vi "Poll Data.vi"(8 "error in":errorcluster, 11 "CR5 in":refnum<class "CR5.lvclass">) -> (0 "error out":errorcluster, 2 "Data Out":refnum<class "Data.lvclass">, 3 "CR5 out":refnum<class "CR5.lvclass">)   [LabVIEW 2015, in "CR5.lvclass"]
doc: "Use this VI when the hygrometer has been set to poll to poll data from the device. The hygrometer is set to poll via commands at boot time."
uses:
  CR5.lvclass
  Reusable/Data/Data.lvclass
  Reusable/Session APIs/Serial/Serial Session.lvclass
  CR5.lvclass/CR5.ctl
  Data/CR5 Data.lvclass
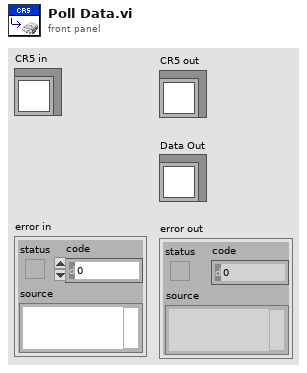
[diagram p1: front panel]
types:
  T1 = typedef "Session - Root.lvclass/Session Handle.ctl" = refnum<data-value>
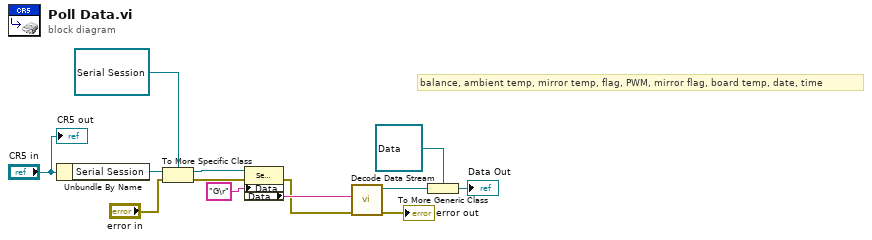
[diagram p0: block diagram]
diagram:
  # "balance, ambient temp, mirror temp, flag, PWM, mirror flag, board temp, date, time"
  n1 = Unbundle By Name("CR5 in") -> ("Serial Session"=w12:T1)
  n2 = To More Specific Class(target class=refnum<data-value> refnum, reference=w12, error in="error in") -> (specific class reference=w10:refnum<data-value>, error out=w9:errorcluster)
  n3 = property class="Serial Session"(reference=w10, error in=w9, "Data"="G\r") -> (error out=w5:errorcluster, "Data"=w6:string)  [unwired: 1 out]
  n4 = call "Decode Data Stream.vi"("error in (no error)"=w5, "string"=w6) -> ("error out"=→"error out":errorcluster, "CR5 Data out"=w3:refnum<class "CR5 Data.lvclass">)  [unwired: 8 in]
  n5 = To More Generic Class(target class=refnum<class "Data.lvclass"> refnum ("Base Data Lib:Data"), reference=w3) -> (generic class reference=→"Data Out":refnum<class "Data.lvclass">)
  "CR5 out" <- "CR5 in"
